vi "Active Option Update.vi"(8 "error in (no error)":errorcluster, 10 "Active Option":string, 11 "Fancy Car Position Simulation View in":refnum<class "Fancy Car Position Simulation View.lvclass">) -> (0 "error out":errorcluster, 3 "Fancy Car Position Simulation View out":refnum<class "Fancy Car Position Simulation View.lvclass">)   [LabVIEW 2019, in "Fancy Car Position Simulation View.lvclass"]
uses:
  <vilib>/gpm_packages/@cs/Car-wash/Source/Fancy Car Position Simulation View/Fancy Car Position Simulation View/Fancy Car Position Simulation View.lvclass
  C:/Program Files/National Instruments/LabVIEW 2019/vi.lib/gpm_packages/@cs/Car-wash/Source/Car Position Simulation View Definition/Car Position Simulation View Definition/Car Position Simulation View Definition.lvclass
  <vilib>/gpm_packages/@cs/Car-wash/Source/Car Position Simulation View Definition/Car Position Simulation View Definition/Car Position Simulation View Definition.lvclass/Car Position Simulation View Definition.ctl
  <vilib>/gpm_packages/@cs/Car-wash/Source/Car Position Simulation View Definition/Car Position Simulation View Definition/Car Position Simulation View Definition.lvclass
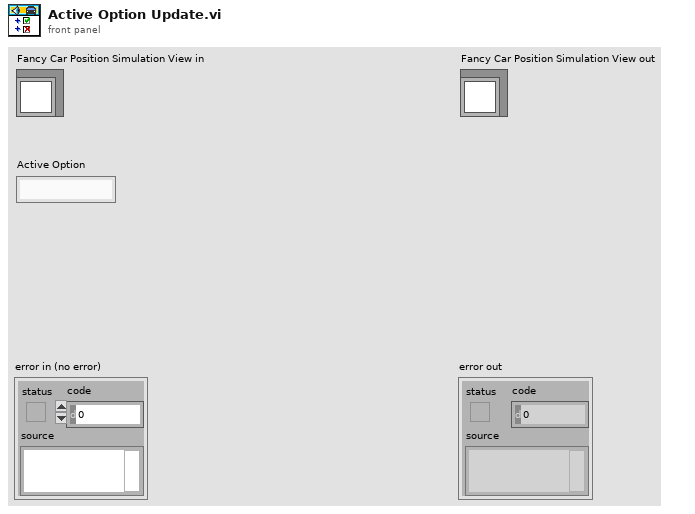
[diagram p1: front panel]
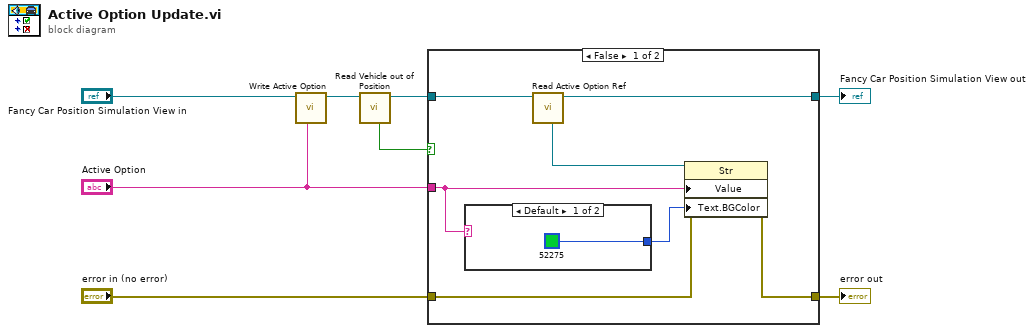
[diagram p0: block diagram]
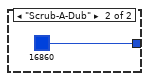
[diagram p2: hidden frame]
diagram:
  n1 = call <vilib>:"Write Active Option.vi"("Active Option"="Active Option", "Car Position Simulation View Definition in"="Fancy Car Position Simulation View in") -> ("Car Position Simulation View Definition out"=w3:refnum<class "Fancy Car Position Simulation View.lvclass">)  [unwired: 9 in]
  n2 = call <vilib>:"Read Vehicle out of Position.vi"("Car Position Simulation View Definition in"=w3) -> ("Car Position Simulation View Definition out"=w2:refnum<class "Fancy Car Position Simulation View.lvclass">, "Vehicle out of Position"=w1:bool)  [unwired: 9 in]
  n3 = case shown="False" w1 {
    tunnel: [w15 w19] -> w8
    tunnel: "error in (no error)" -> [w13 w18]
    tunnel: [w12 w18] -> w6
    tunnel: "Active Option" -> [w10 _]
    tunnel: w2 -> [w9 w19]
    frame False {
      n4 = case shown="Default" w10 {
        tunnel: [u32 52275 u32 16860] -> w11
        frame Default {
        }
        frame "Scrub-A-Dub" {
        }
      }
      n5 = call <vilib>:"Read Active Option Ref.vi"("Car Position Simulation View Definition in"=w9) -> ("Car Position Simulation View Definition out"=w15:refnum<class "Fancy Car Position Simulation View.lvclass">, "Active Option Ref"=w14:refnum<vi>)  [unwired: 9 in]
      n6 = property class="Str"(reference=w14, error in=w13, "Value"=w10, "Text.BGColor"=w11) -> (error out=w12:errorcluster)  [unwired: 1 out]
    }
    frame True {
    }
  }
  "error out" <- w6
  "Fancy Car Position Simulation View out" <- w8
